vi "ZDataVIS_Extract_Value_from_Patrick's_YAML.vi"(11 "String":string) -> (3 "Numeric":dbl)   [LabVIEW 2016]
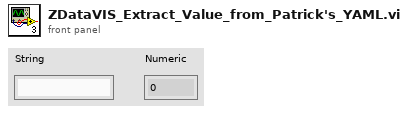
[diagram p1: front panel]
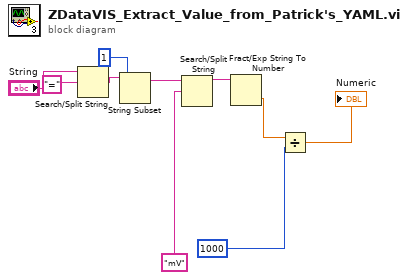
[diagram p0: block diagram]
diagram:
  n1 = Search/Split String(string="String", search string/char (-)="=") -> (match + rest of string=w5:string)  [unwired: 1 in, 2 out]
  n2 = String Subset(string=w5, offset (0)=1) -> (substring=w7:string)  [unwired: 1 in]
  n3 = Search/Split String(string=w7, search string/char (-)="mV") -> (substring before match=w6:string)  [unwired: 1 in, 2 out]
  n4 = Fract/Exp String To Number(string=w6) -> (number=w2:dbl)  [unwired: 3 in, 1 out]
  n5 = Divide(x=w2, y=1000) -> (x/y=→"Numeric":dbl)
